vi "GetDiagramUIDs.vi"(6 "error in":errorcluster, 9 "FlatSequenceFrame in":refnum<class "FlatSequenceFrame.lvclass">) -> (0 "error out":errorcluster, 3 "FlatSequenceFrame out":refnum<class "FlatSequenceFrame.lvclass">, 4 "diagrams":i32[](array[numeric]))   [LabVIEW 2014, in "Raspberry Pi Compatible Compiler for LabVIEW.lvlib" / "FlatSequenceFrame.lvclass"]
uses:
  FlatSequenceFrame.lvclass
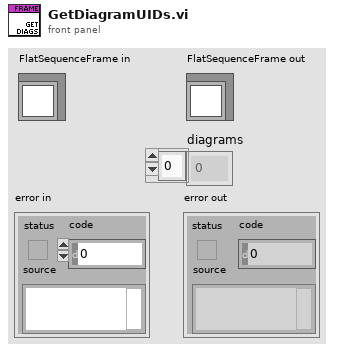
[diagram p1: front panel]
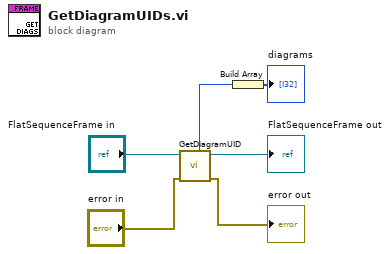
[diagram p0: block diagram]
diagram:
  n1 = call-dynamic "GetDiagramUID.vi"("error in"="error in", "FlatSequenceFrame in"="FlatSequenceFrame in") -> ("error out"=→"error out":errorcluster, "FlatSequenceFrame out"=→"FlatSequenceFrame out":refnum<class "FlatSequenceFrame.lvclass">, "Diagram.UID"=w2:i32)  [unwired: 5 in]
  n2 = Build Array(w2) -> (→"diagrams":i32[])
